vi "XML Loop Stack Recursion.vi"(8 "error in":errorcluster, 9 "type":variant, 10 "xml string":string) -> (0 "error out":errorcluster, 2 "data out":variant)   [LabVIEW 2013]
uses:
  Support/Type Defs/Formatting Data Type -- Enum.ctl
  <userlib>/_OpenG.lib/array/array.llb/Conditional Auto-Indexing Tunnel (I32)__ogtk.vi
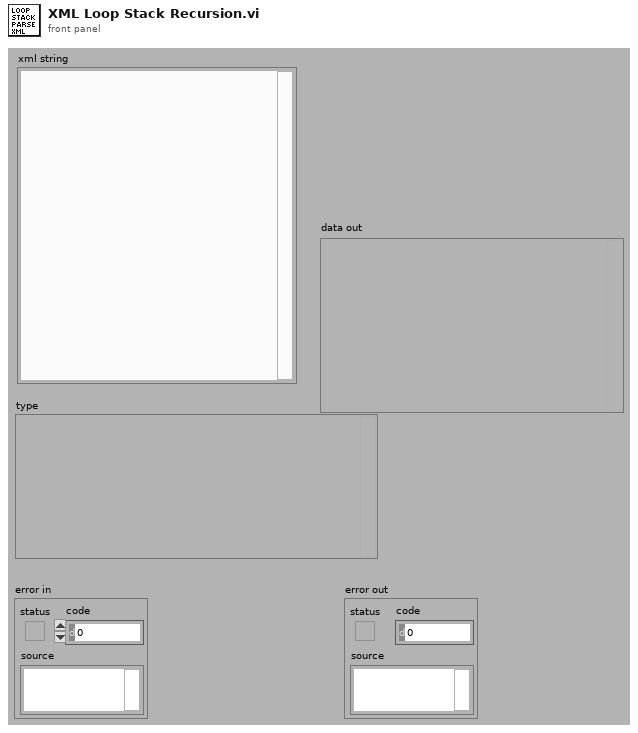
[diagram p1: front panel]
types:
  T1 = typedef "Formatting Data Type -- Enum.ctl" = enum16{"<unknown>", "Cluster", "Array", "String", "Path", "Boolean", "Time Stamp", "Enum", "Numeric - EXT", "Numeric - DBL", "Numeric - SGL", "Numeric - I64", "Numeric - I32", "Numeric - I16", "Numeric - I8", "Numeric - U64", "Numeric - U32", "Numeric - U16", "Numeric - U8", "Numeric - CXT", "Numeric - CDB", "Numeric - CSG", "VISA Resource"}
  T2 = cluster{"xml index":i32, "level":i32, "dup Data":variant, "attribute":bool, "EasyXML Type":T1, "treated xml name":string, "attributes cluster?":bool, "untreated Data Name":string, "parent name":string, "Parent Type":T1, "pretty print level":i32}
  T3 = typedef "XML Structure - Cluster.ctl" = cluster{"tags":string[], "tag names":string[], "tag type":T4[], "offset":i32[], "close tag index":i32[], "xml":string, "Children":cluster{"children":i32[]}[], "parent index":i32[]}
  T4 = typedef "XML Tag Type - Enum.ctl" = enum16{"start tag", "empty tag", "end tag"}
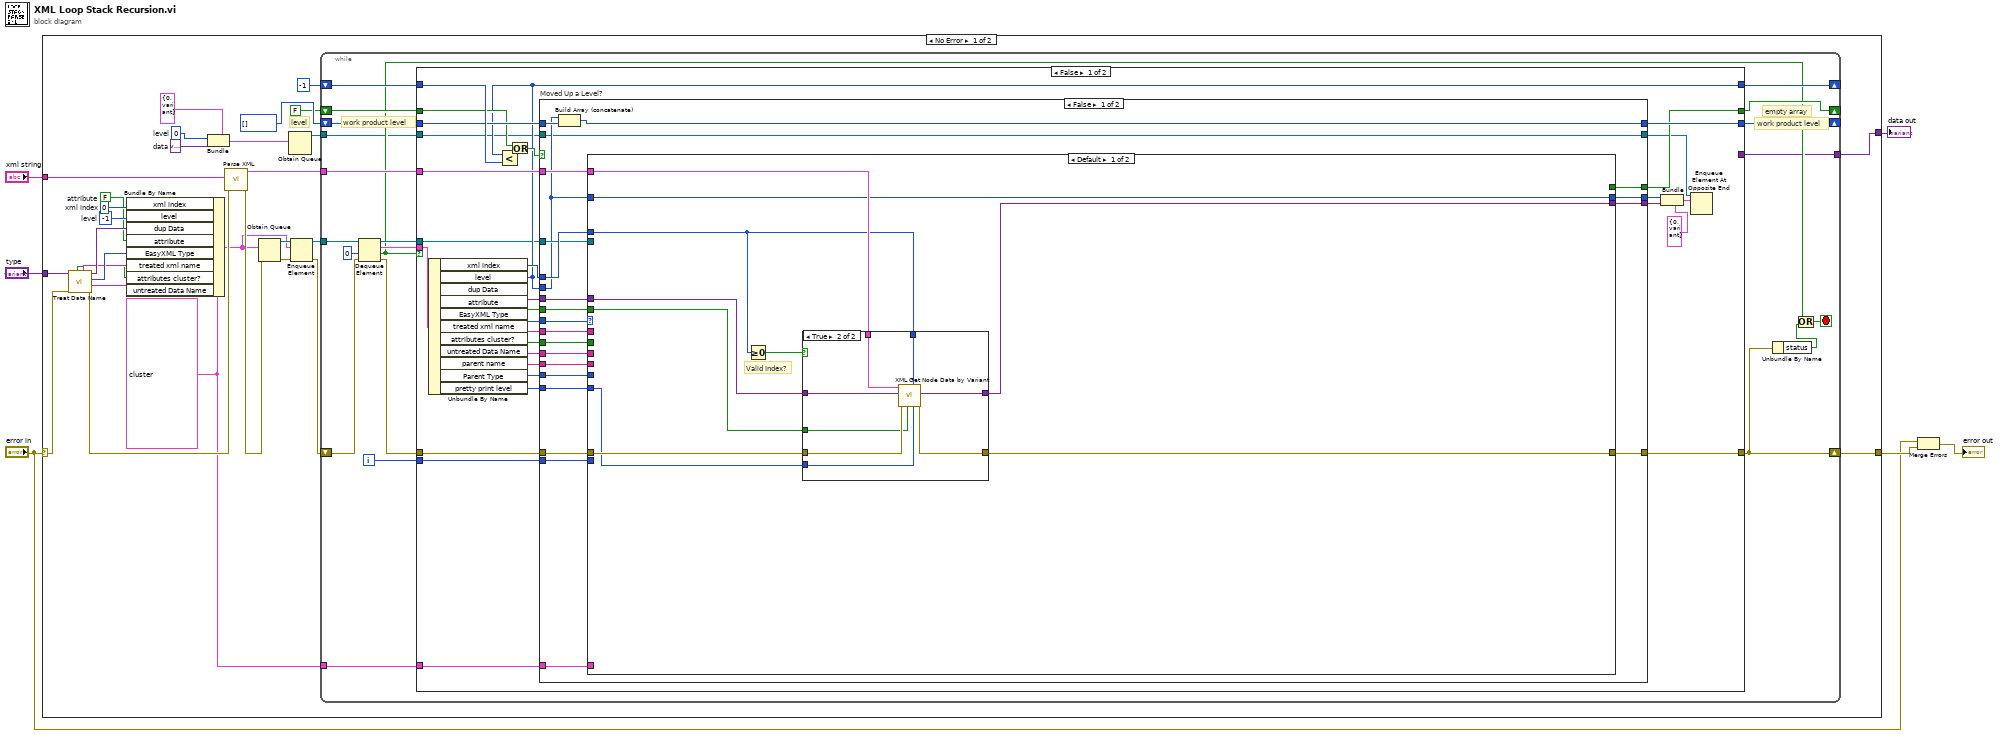
[diagram p0: block diagram]
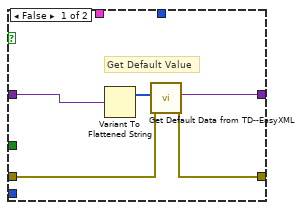
[diagram p2: hidden frame]
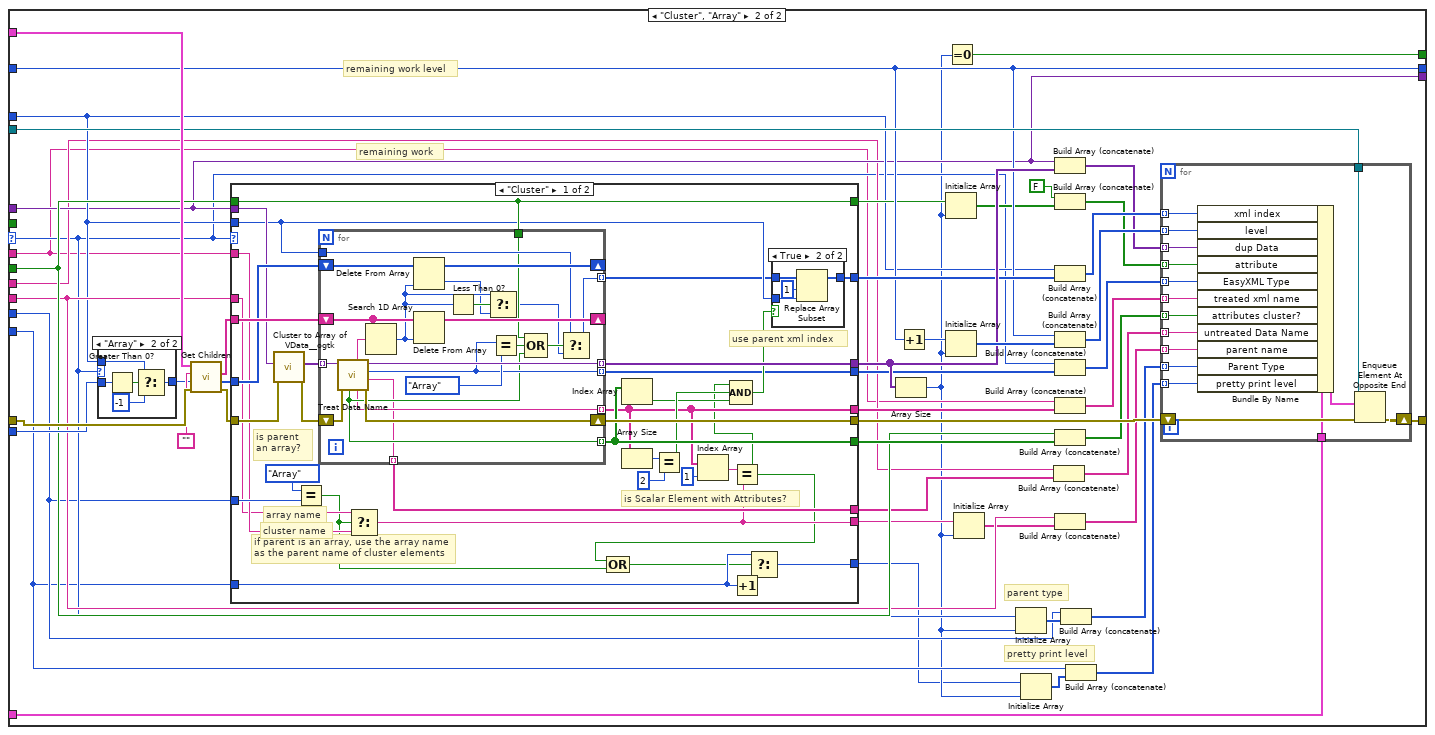
[diagram p3: hidden frame]
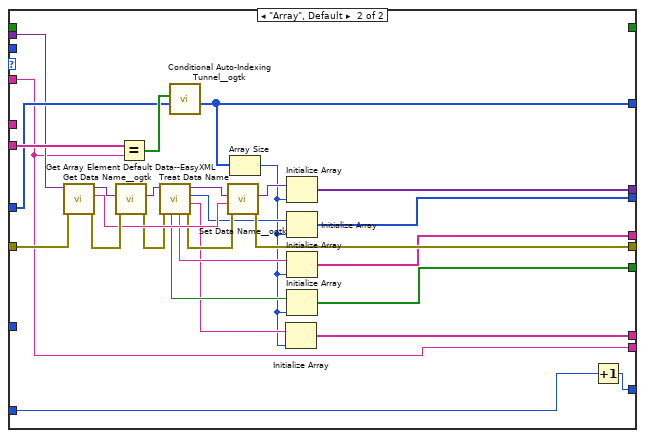
[diagram p6: hidden frame]
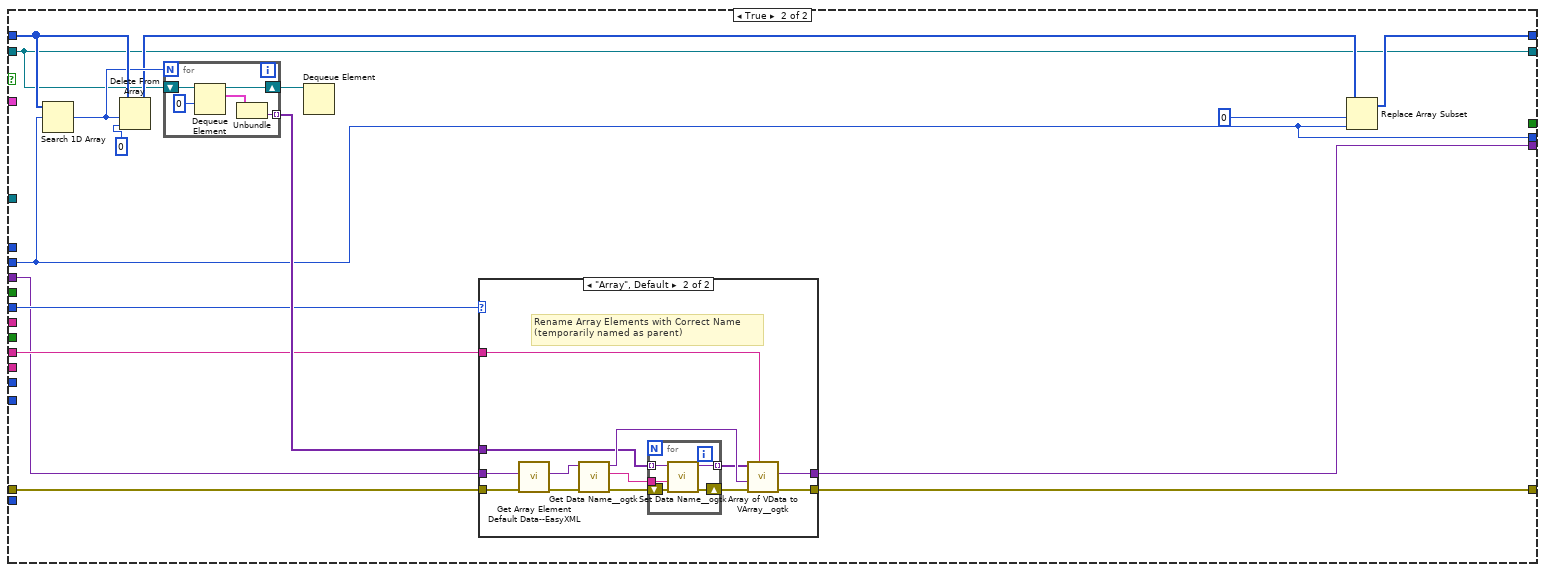
[diagram p7: hidden frame]
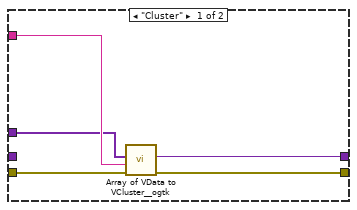
[diagram p8: hidden frame]
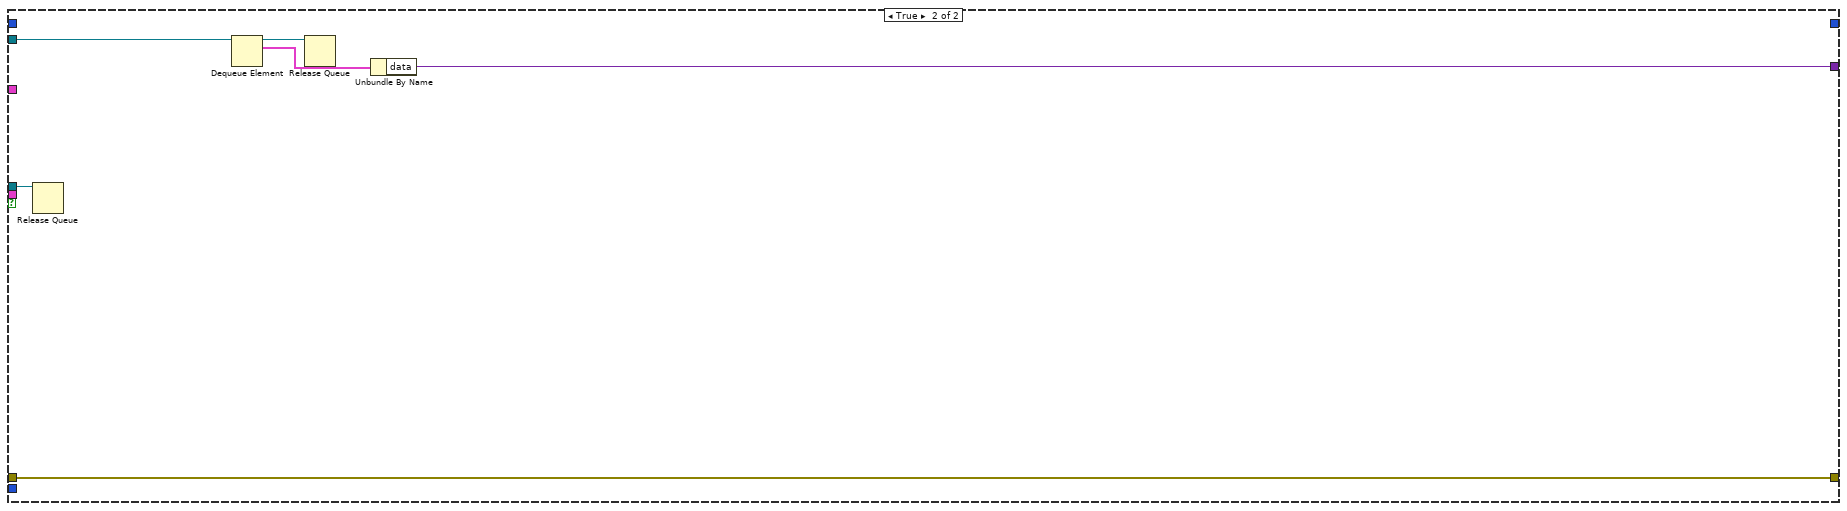
[diagram p9: hidden frame]
diagram:
  n1 = case shown="No Error" "error in" {
    selector: "error in" -> [w19 w347]
    tunnel: [w21 _] -> w6
    tunnel: "xml string" -> [w34 _]
    tunnel: "type" -> [w20 _]
    tunnel: [w32 w347] -> w2
    frame No Error {
      w7 = T2 {"xml index"=0, "level"=0, "dup Data"=variant, "attribute"=FALSE, "EasyXML Type"=enum."<unknown>", "treated xml name"="", "attributes cluster?"=FALSE, "untreated Data Name"="", "parent name"="", "Parent Type"=enum."<unknown>", "pretty print level"=0} ("cluster")
      w23 = variant  # data
      w13 = FALSE  # attribute
      w24 = 0  # level
      w16 = 0  # xml index
      w15 = -1  # level
      # "level"
      n2 = call "Treat Data Name.vi"("error in (no error)"=w19, "Data"=w20) -> ("error out"=w18:errorcluster, "untreated Data Name"=w9:string, "EasyXML Type"=w12:T1, "dup Data"=w14:variant, "treated xml name"=w11:string, "attributes cluster?"=w10:bool)  [unwired: 3 in, 1 out]
      n3 = Bundle By Name(cluster=w7, "xml index"=w16, "level"=w15, "dup Data"=w14, "attribute"=w13, "EasyXML Type"=w12, "treated xml name"=w11, "attributes cluster?"=w10, "untreated Data Name"=w9) -> (w8:T2)
      n4 = Bundle(cluster=cluster{"level":i32, "data":variant} {"level"=0, "data"=variant}, "level"=w24, "data"=w23) -> (w25:cluster{"level":i32, "data":variant})
      n5 = call "Parse XML.vi"("error in (no error)"=w18, "xml string"=w34) -> ("error out"=w27:errorcluster, "xml out"=w33:T3)  [unwired: 8 in]
      n6 = Obtain Queue(element data type=w8, error in (no error)=w27) -> (queue out=w30:refnum<queue>, error out=w28:errorcluster)  [unwired: 3 in, 1 out]
      n7 = Obtain Queue(element data type=w25) -> (queue out=w22:refnum<queue>)  [unwired: 4 in, 2 out]
      n8 = Enqueue Element(queue=w30, element=w8, error in (no error)=w28) -> (queue out=w29:refnum<queue>, error out=w26:errorcluster)  [unwired: 1 in, 1 out]
      n9 = while {
        shift-right: [w50] -> w32
        shift-left: w26 -> [w41]
        shift-right: [w55] -> _
        shift-left: i32[] [] -> [w56]
        shift-right: [w44] -> _
        shift-left: -1 -> [w57]
        tunnel: w33 -> [w54]
        shift-right: [w53] -> _
        shift-left: FALSE -> [w52]
        tunnel: w29 -> [w47]
        tunnel: w22 -> [w39]
        tunnel: [w38] -> w21
        tunnel: w7 -> [w37]
        i -> [w51]
        stop <- w48 stop-if-true
        # "empty array"
        # "work product level"
        # "work product level"
        n10 = Dequeue Element(queue=w47, timeout in ms (-1)=0, error in (no error)=w41) -> (queue out=w43:refnum<queue>, element=w45:T2, timed out?=w42:bool, error out=w40:errorcluster)
        n11 = case shown="False" w42 {
          tunnel: w57 -> [w88 _]
          tunnel: w56 -> [w87 _]
          tunnel: w40 -> [w86 w345]
          tunnel: [w85 _] -> w55
          tunnel: w54 -> [w84 _]
          tunnel: [w83 _] -> w53
          tunnel: w52 -> [w82 _]
          tunnel: w51 -> [w79 _]
          tunnel: [w78 w345] -> w50
          tunnel: w45 -> [w77 _]
          tunnel: [w75 _] -> w44
          tunnel: w43 -> [w73 w346]
          tunnel: w39 -> [w61 w344]
          tunnel: [_ w341] -> w38
          tunnel: w37 -> [w58 _]
          frame False {
            n12 = Unbundle By Name(w77) -> ("xml index"=w76:i32, "level"=w75:i32, "dup Data"=w74:variant, "attribute"=w69:bool, "EasyXML Type"=w68:T1, "treated xml name"=w67:string, "attributes cluster?"=w66:bool, "untreated Data Name"=w65:string, "parent name"=w63:string, "Parent Type"=w62:T1, "pretty print level"=w59:i32)
            n13 = Less?(x=w75, y=w88) -> (x < y?=w81:bool)
            n14 = Or(x=w82, y=w81) -> (x .or. y?=w80:bool)
            n15 = case "Moved Up a Level?" shown="False" w80 {
              tunnel: w87 -> [w94 w311]
              tunnel: [w92 w305] -> w85
              tunnel: [w111 w312] -> w78
              tunnel: w86 -> [w98 w299]
              tunnel: w74 -> [w99 w298]
              tunnel: w75 -> [w93 w303]
              tunnel: w84 -> [w110 _]
              tunnel: w76 -> [w109 _]
              tunnel: [w108 _] -> w83
              tunnel: w79 -> [w107 _]
              tunnel: w73 -> [w106 _]
              tunnel: w61 -> [w91 w297]
              tunnel: [w105 w307] -> w70
              tunnel: [w104 w303] -> w72
              tunnel: w69 -> [w103 _]
              tunnel: w68 -> [w102 w301]
              tunnel: w67 -> [w101 _]
              tunnel: w66 -> [w100 _]
              tunnel: w65 -> [w97 w300]
              tunnel: w63 -> [w96 _]
              tunnel: w62 -> [w95 _]
              tunnel: [w91 w297] -> w60
              tunnel: w59 -> [w90 _]
              tunnel: w58 -> [w89 _]
              frame False {
                n16 = Build Array (concatenate)(w93, w94) -> (w92:i32[])
                n17 = case shown="Default" w102 {
                  selector: w102 -> [_ w144]
                  tunnel: w98 -> [w118 w178]
                  tunnel: [w121 w167] -> w111
                  tunnel: w99 -> [w119 w149]
                  tunnel: w93 -> [w112 w166]
                  tunnel: w110 -> [w120 w182]
                  tunnel: w109 -> [w115 w150]
                  tunnel: [_ w175] -> w108
                  tunnel: w107 -> [_ w174]
                  tunnel: w106 -> [_ w172]
                  tunnel: [w112 w166] -> w104
                  tunnel: [w117 w149] -> w105
                  tunnel: w103 -> [w116 _]
                  tunnel: w100 -> [_ w157]
                  tunnel: w101 -> [_ w143]
                  tunnel: w97 -> [_ w147]
                  tunnel: w96 -> [_ w151]
                  tunnel: w95 -> [_ w141]
                  tunnel: w90 -> [w113 w140]
                  tunnel: w89 -> [_ w135]
                  frame Default {
                    # "Valid Index?"
                    n18 = Greater Or Equal To 0?(x=w115) -> (x >= 0?=w114:bool)
                    n19 = case shown="True" w114 {
                      tunnel: [w123 w134] -> w121
                      tunnel: w120 -> [_ w133]
                      tunnel: w119 -> [w126 w132]
                      tunnel: w118 -> [w124 w131]
                      tunnel: [w122 w130] -> w117
                      tunnel: w116 -> [_ w129]
                      tunnel: w115 -> [_ w128]
                      tunnel: w113 -> [_ w127]
                      frame False {
                        # "Get Default Value"
                        n20 = Variant To Flattened String(Variant=w126) -> (1:w125:i16[])  [unwired: 1 out]
                        n21 = call "Get Default Data from TD--EasyXML.vi"("error in"=w124, "Type Descriptor"=w125) -> ("error out"=w123:errorcluster, "Default VData"=w122:variant)  [unwired: 8 in]
                      }
                      frame True {
                        n22 = call "XML Get Node Data by Variant.vi"("level"=w127, "element id"=w128, "Attribute?(F=Entity)"=w129, "error in (no error)"=w131, "Variant in (type and name)"=w132, "xml"=w133) -> ("error out"=w134:errorcluster, "Variant out"=w130:variant)  [unwired: 4 in]
                      }
                    }
                  }
                  frame "Cluster", "Array" {
                    # "parent type"
                    # "pretty print level"
                    # "remaining work level"
                    # "remaining work"
                    n23 = case shown="\"Array\"" w144 {
                      tunnel: w174 -> [_ w207]
                      tunnel: w150 -> [w202 w205]
                      tunnel: [w202 w204] -> w173
                      frame Default {
                      }
                      frame "Array" {
                        n24 = Greater Than 0?(x=w207) -> (x > 0?=w206:bool)
                        n25 = Select(t=w205, s=w206, f=-1) -> (s? t:f=w204:i32)
                      }
                    }
                    n26 = call "Get Children.vi"("error in (no error)"=w178, "tag index"=w173, "child name (\"\": all children)"="", "xml structure in"=w182) -> ("error out"=w177:errorcluster, "child indices"=w180:i32[], "child names"=w181:string[])  [unwired: 4 in, 1 out]
                    n27 = case shown="\"Cluster\"" w144 {
                      tunnel: [w241 w296] -> w168
                      tunnel: w149 -> [w234 w286]
                      tunnel: [w236 w294] -> w183
                      tunnel: w150 -> [w222 _]
                      tunnel: w181 -> [w238 w289]
                      tunnel: w180 -> [w237 w288]
                      tunnel: [w219 w287] -> w179
                      tunnel: w177 -> [w233 w285]
                      tunnel: [w235 _] -> w165
                      tunnel: w157 -> [w235 _]
                      tunnel: w143 -> [w216 w271]
                      tunnel: [w221 w279] -> w160
                      tunnel: [w226 w277] -> w155
                      tunnel: [w231 w275] -> w158
                      tunnel: [w232 w272] -> w154
                      tunnel: w151 -> [w215 _]
                      tunnel: [w214 w271] -> w142
                      tunnel: w141 -> [w217 _]
                      tunnel: w140 -> [w213 w269]
                      tunnel: [w211 w270] -> w138
                      frame "Cluster" {
                        # "if parent is an array, use the array name as the parent name of cluster elements"
                        # "array name"
                        # "cluster name"
                        # "is parent an array?"
                        # "use parent xml index"
                        # "is Scalar Element with Attributes?"
                        n28 = call <userlib>:"Cluster to Array of VData__ogtk.vi"("error in (no error)"=w233, "Cluster"=w234) -> ("error out"=w240:errorcluster, "Array of VData"=w239:variant[])  [unwired: 8 in]
                        n29 = Equal?(x=Formatting_Data_Type_--_Enum."Array" ("EasyXML Type"), y=w217) -> (x = y?=w210:bool)
                        n30 = for {
                          shift-right: [w266] -> w241
                          shift-left: w240 -> [w267]
                          tunnel: w239 -> [w268] mode=indexing
                          shift-right: [w264] -> _
                          shift-left: w238 -> [w265]
                          shift-right: [w262] -> _
                          shift-left: w237 -> [w263]
                          tunnel: [w256] -> w220 mode=indexing
                          tunnel: [w261] -> w236 mode=indexing
                          tunnel: w222 -> [w260]
                          tunnel: w235 -> [w258]
                          tunnel: [w250] -> w221 mode=indexing
                          tunnel: [w249] -> w231 mode=indexing
                          tunnel: [w248] -> w226 mode=indexing
                          tunnel: [w247] -> w232 mode=indexing
                          n31 = call "Treat Data Name.vi"("error in (no error)"=w267, "Data"=w268) -> ("error out"=w266:errorcluster, "untreated Data Name"=w247:string, "EasyXML Type"=w250:T1, "dup Data"=w261:variant, "treated xml name"=w248:string, "attributes cluster?"=w249:bool)  [unwired: 3 in, 1 out]
                          n32 = Search 1D Array(1D array=w265, element=w248) -> (index of element=w254:i32)  [unwired: 1 in]
                          n33 = Delete From Array(array=w263, index=w254) -> (deleted portion=w253:i32, array with subset deleted=w262:i32[])  [unwired: 1 in]
                          n34 = Delete From Array(array=w265, index=w254) -> (array with subset deleted=w264:string[])  [unwired: 1 in, 1 out]
                          n35 = Less Than 0?(x=w254) -> (x < 0?=w255:bool)
                          n36 = Select(t=w254, s=w255, f=w253) -> (s? t:f=w252:i32)
                          n37 = Equal?(x=w250, y=Formatting_Data_Type_--_Enum."Array" ("EasyXML Type")) -> (x = y?=w259:bool)
                          n38 = Compound Arithmetic op=OR(w258, w259, w249) -> (w257:bool)
                          n39 = Select(t=w260, s=w257, f=w252) -> (s? t:f=w256:i32)
                        }
                        n40 = Select(t=w215, s=w210, f=w216) -> (s? t:f=w214:string)
                        n41 = Index Array(array=w231) -> (element=w227:bool)  [unwired: 1 in]
                        n42 = Array Size(array=w226) -> (size(s)=w230:i32)
                        n43 = Equal?(x=w230, y=2 ("x")) -> (x = y?=w228:bool)
                        n44 = Index Array(array=w226, index=1) -> (element=w224:string)
                        n45 = Equal?(x=w224, y=w214) -> (x = y?=w209:bool)
                        n46 = Compound Arithmetic op=OR(w209, w210) -> (w208:bool)
                        n47 = Compound Arithmetic op=AND(w209, w228, w227) -> (w223:bool)
                        n48 = Increment(x=w213) -> (x+1=w212:i32)
                        n49 = Select(t=w213, s=w208, f=w212) -> (s? t:f=w211:i32)
                        n50 = case shown="True" w223 {
                          tunnel: w220 -> [w242 w246]
                          tunnel: [w242 w245] -> w219
                          tunnel: w222 -> [_ w244]
                          frame False {
                          }
                          frame True {
                            n51 = Replace Array Subset(array=w246, new element=w244, index=1) -> (w245:i32[])
                          }
                        }
                      }
                      frame "Array", Default {
                        n52 = call <userlib>:"Get Data Name__ogtk.vi"("error in (no error)"=w285, "Data"=w286) -> ("error out"=w292:errorcluster, "Data Name"=w291:string, "Data dup"=w293:variant)  [unwired: 7 in]
                        n53 = call "Get Array Element Default Data--EasyXML.vi"("error in (no error)"=w292, "Array"=w293) -> ("error out"=w281:errorcluster, "Array Element Default Data"=w284:variant)  [unwired: 8 in]
                        n54 = Equal?(x=w289, y=w271) -> (x = y?=w290:bool[])
                        n55 = call "Treat Data Name.vi"("error in (no error)"=w281, "Data"=w284) -> ("error out"=w282:errorcluster, "untreated Data Name"=w274:string, "EasyXML Type"=w280:T1, "dup Data"=w283:variant, "treated xml name"=w278:string, "attributes cluster?"=w276:bool)  [unwired: 3 in, 1 out]
                        n56 = call-poly <userlib>:"Conditional Auto-Indexing Tunnel__ogtk.vi"("Array in"=w288, "Elements to keep"=w290) -> ("Filtered Array out"=w287:i32[])  [unwired: 5 in]
                        n57 = call <userlib>:"Set Data Name__ogtk.vi"("error in (no error)"=w282, "Data Name"=w291, "Data"=w283) -> ("error out"=w296:errorcluster, "Renamed Data"=w295:variant)  [unwired: 7 in]
                        n58 = Array Size(array=w287) -> (size(s)=w273:i32)
                        n59 = Initialize Array(w274, w273) -> (w272:string[])
                        n60 = Initialize Array(w295, w273) -> (w294:variant[])
                        n61 = Initialize Array(w280, w273) -> (w279:T1[])
                        n62 = Initialize Array(w278, w273) -> (w277:string[])
                        n63 = Initialize Array(w276, w273) -> (w275:bool[])
                        n64 = Increment(x=w269) -> (x+1=w270:i32)
                      }
                    }
                    n65 = Array Size(array=w183) -> (size(s)=w139:i32)
                    n66 = Increment(x=w166) -> (x+1=w185:i32)
                    n67 = Initialize Array(w165, w139) -> (w164:bool[])
                    n68 = Initialize Array(w185, w139) -> (w184:i32[])
                    n69 = Equal To 0?(x=w139) -> (x = 0?=w175:bool)
                    n70 = Initialize Array(w142, w139) -> (w148:string[])
                    n71 = Initialize Array(w144, w139) -> (w145:T1[])
                    n72 = Initialize Array(w138, w139) -> (w137:i32[])
                    n73 = Build Array (concatenate)(w147, w154) -> (w153:string[])
                    n74 = Build Array (concatenate)(w149, w183) -> (w169:variant[])
                    n75 = Build Array (concatenate)(FALSE, w164) -> (w162:bool[])
                    n76 = Build Array (concatenate)(w150, w179) -> (w171:i32[])
                    n77 = Build Array (concatenate)(w166, w184) -> (w170:i32[])
                    n78 = Build Array (concatenate)(w144, w160) -> (w161:T1[])
                    n79 = Build Array (concatenate)(w143, w155) -> (w156:string[])
                    n80 = Build Array (concatenate)(w157, w158) -> (w159:bool[])
                    n81 = Build Array (concatenate)(w151, w148) -> (w152:string[])
                    n82 = Build Array (concatenate)(w141, w145) -> (w146:T1[])
                    n83 = Build Array (concatenate)(w140, w137) -> (w136:i32[])
                    n84 = for {
                      tunnel: w172 -> [w201]
                      tunnel: w171 -> [w199] mode=indexing
                      tunnel: w170 -> [w198] mode=indexing
                      tunnel: w169 -> [w197] mode=indexing
                      shift-right: [w195] -> w167
                      shift-left: w168 -> [w196]
                      tunnel: w162 -> [w194] mode=indexing
                      tunnel: w161 -> [w193] mode=indexing
                      tunnel: w156 -> [w192] mode=indexing
                      tunnel: w159 -> [w191] mode=indexing
                      tunnel: w153 -> [w190] mode=indexing
                      tunnel: w135 -> [w189]
                      tunnel: w152 -> [w188] mode=indexing
                      tunnel: w146 -> [w187] mode=indexing
                      tunnel: w136 -> [w186] mode=indexing
                      n85 = Bundle By Name(cluster=w189, "xml index"=w199, "level"=w198, "dup Data"=w197, "attribute"=w194, "EasyXML Type"=w193, "treated xml name"=w192, "attributes cluster?"=w191, "untreated Data Name"=w190, "parent name"=w188, "Parent Type"=w187, "pretty print level"=w186) -> (w200:T2)
                      n86 = Enqueue Element At Opposite End(queue=w201, element=w200, error in (no error)=w196) -> (error out=w195:errorcluster)  [unwired: 1 in, 2 out]
                    }
                  }
                }
              }
              frame True {
                n87 = Search 1D Array(1D array=w311, element=w303) -> (index of element=w309:i32)  [unwired: 1 in]
                n88 = Delete From Array(array=w311, length=w309, index=0) -> (array with subset deleted=w306:i32[])  [unwired: 1 out]
                n89 = for {
                  N: w309 -> [_]
                  tunnel: [w314] -> w308 mode=indexing
                  shift-right: [w313] -> w302
                  shift-left: w297 -> [w316]
                  n90 = Dequeue Element(queue=w316, timeout in ms (-1)=0) -> (queue out=w313:refnum<queue>, element=w315:cluster{"level":i32, "data":variant})  [unwired: 1 in, 2 out]
                  n91 = Unbundle(w315) -> ("data"=w314:variant)  [unwired: 1 out]
                }
                n92 = Dequeue Element(queue=w302) -> ()  [unwired: 2 in, 4 out]
                n93 = case shown="\"Array\", Default" w301 {
                  tunnel: w300 -> [w322 w335]
                  tunnel: [w321 w334] -> w307
                  tunnel: [w320 w333] -> w312
                  tunnel: w299 -> [w319 w331]
                  tunnel: w308 -> [w318 w327]
                  tunnel: w298 -> [_ w332]
                  frame "Cluster" {
                    n94 = call <userlib>:"Array of VData to VCluster__ogtk.vi"("error in (no error)"=w319, "Cluster Name"=w322, "Array"=w318) -> ("error out"=w320:errorcluster, "VCluster"=w321:variant)  [unwired: 7 in]
                  }
                  frame "Array", Default {
                    # "Rename Array Elements with Correct Name\n(temporarily named as parent)"
                    n95 = call "Get Array Element Default Data--EasyXML.vi"("error in (no error)"=w331, "Array"=w332) -> ("error out"=w328:errorcluster, "Array Element Default Data"=w330:variant)  [unwired: 8 in]
                    n96 = call <userlib>:"Get Data Name__ogtk.vi"("error in (no error)"=w328, "Data"=w330) -> ("error out"=w325:errorcluster, "Data Name"=w323:string, "Data dup"=w329:variant)  [unwired: 7 in]
                    n97 = for {
                      tunnel: w327 -> [w340] mode=indexing
                      tunnel: [w339] -> w326 mode=indexing
                      shift-right: [w338] -> w324
                      shift-left: w325 -> [w337]
                      tunnel: w323 -> [w336]
                      n98 = call <userlib>:"Set Data Name__ogtk.vi"("error in (no error)"=w337, "Data Name"=w336, "Data"=w340) -> ("error out"=w338:errorcluster, "Renamed Data"=w339:variant)  [unwired: 7 in]
                    }
                    n99 = call <userlib>:"Array of VData to VArray__ogtk.vi"("Array Name"=w335, "error in (no error)"=w324, "Element Type (when empty)"=w329, "1D Array of VData"=w326) -> ("error out"=w333:errorcluster, "VArray"=w334:variant)  [unwired: 6 in]
                  }
                }
                n100 = Replace Array Subset(array=w306, new element=w303, index=0) -> (w305:i32[])
              }
            }
            n101 = Bundle(cluster=cluster{"level":i32, variant} {"level"=0, variant}, "level"=w72, w70) -> (w71:cluster{"level":i32, variant})
            n102 = Enqueue Element At Opposite End(queue=w60, element=w71) -> ()  [unwired: 2 in, 3 out]
          }
          frame True {
            n103 = Release Queue(queue=w346) -> ()  [unwired: 2 in, 3 out]
            n104 = Dequeue Element(queue=w344) -> (queue out=w343:refnum<queue>, element=w342:cluster{"level":i32, "data":variant})  [unwired: 2 in, 2 out]
            n105 = Release Queue(queue=w343) -> ()  [unwired: 2 in, 3 out]
            n106 = Unbundle By Name(w342) -> ("data"=w341:variant)
          }
        }
        n107 = Unbundle By Name(w50) -> ("status"=w49:bool)
        n108 = Or(x=w42, y=w49) -> (x .or. y?=w48:bool)
      }
    }
    frame Error {
    }
  }
  "data out" <- w6
  n109 = Merge Errors("error in", w2) -> (→"error out":errorcluster)
